vi "JKISM++ Post Message.vi"(8 "Error In (no error)":errorcluster, 9 "Dest Module":string="A", 10 "Arguments (\"\")":string, 11 "States":string="DoA") -> (0 "error IO":errorcluster)   [LabVIEW 2014, in "JKI-State-Machine-Plus.lvlib"]
uses:
  JKI-State-Machine-Plus.lvlib
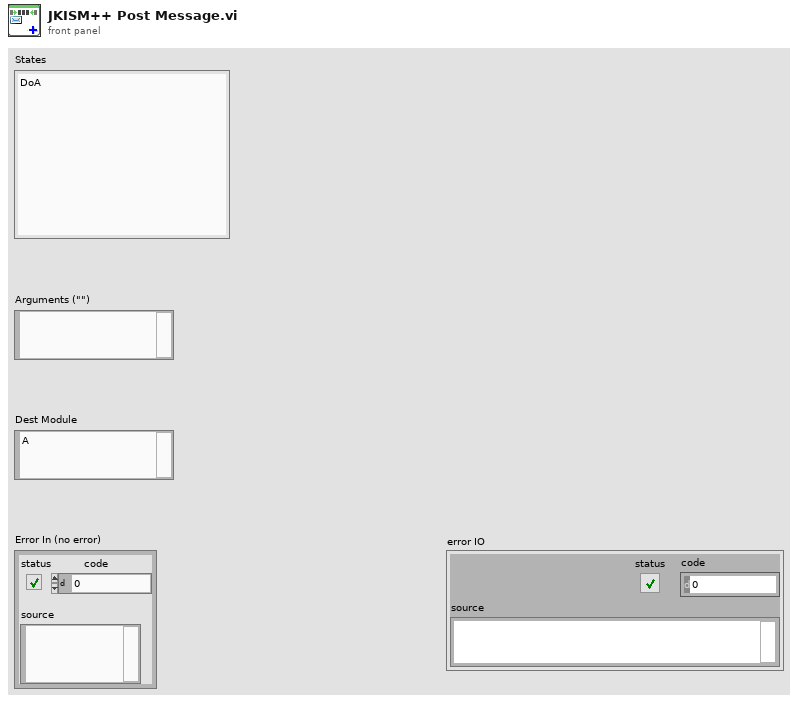
[diagram p1: front panel]
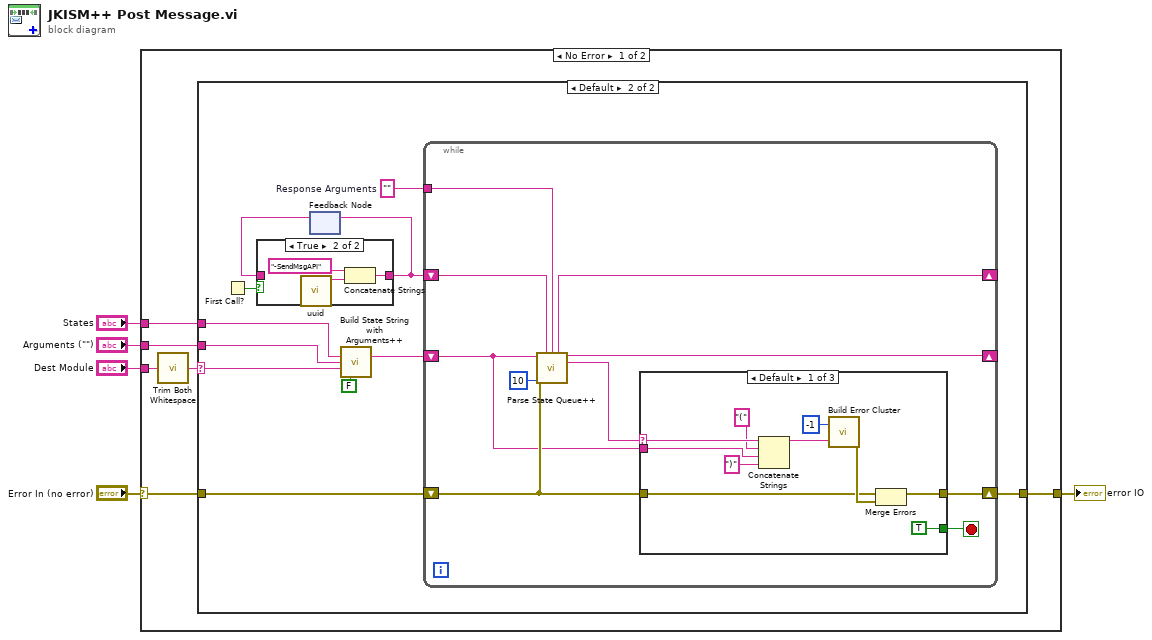
[diagram p0: block diagram]
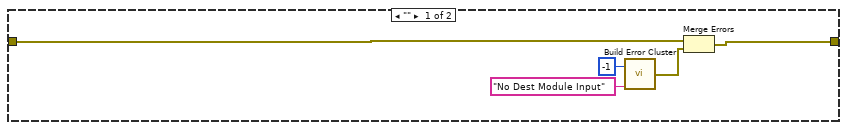
[diagram p2: hidden frame]
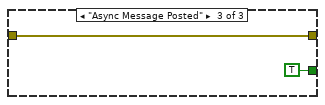
[diagram p5: hidden frame]
diagram:
  n1 = case shown="No Error" "Error In (no error)" {
    selector: "Error In (no error)" -> [w7 w55]
    tunnel: "States" -> [w11 _]
    tunnel: [w8 w55] -> w3
    tunnel: "Arguments (\"\")" -> [w10 _]
    tunnel: "Dest Module" -> [w9 _]
    frame No Error {
      n2 = call "Trim Both Whitespace.vi"("string"=w9) -> ("trimmed string"=w6:string)  [unwired: 1 in]
      n3 = case shown="Default" w6 {
        selector: w6 -> [_ w25]
        tunnel: w11 -> [_ w27]
        tunnel: w10 -> [_ w26]
        tunnel: [w15 w22] -> w8
        tunnel: w7 -> [w16 w21]
        frame "" {
          n4 = call "Build Error Cluster.vi"("String to Prepend to source (\"\")"="No Dest Module Input" ("String to Prepend to source (\"\")"), "code"=-1) -> ("error out"=w14:errorcluster)
          n5 = Merge Errors(w16, w14) -> (w15:errorcluster)
        }
        frame Default {
          w23 = ""  # Response Arguments
          n6 = First Call?() -> (First Call?: T/F=w19:bool)
          n7 = feedback #1() -> (w18:string)  [unwired: 1 in]
          n8 = case shown="True" w19 {
            tunnel: [w28 w29] -> w17
            tunnel: w18 -> [w28 _]
            frame False {
            }
            frame True {
              n9 = call "uuid.vi"() -> ("UUID"=w30:string)  [unwired: 11 in]
              n10 = Concatenate Strings("-SendMsgAPI" ("Name(\"\" to use uuid)"), w30) -> (w29:string)
            }
          }
          n11 = feedback-in #1(w17) -> ()
          n12 = call "Build State String with Arguments++.vi"("State"=w27, "Arguments (\"\")"=w26, "Dest Module (\"\")"=w25, "Sync-Call(@) T By Default/Async-Call(->) F"=FALSE) -> ("State with Arguments"=w20:string)  [unwired: 11 in]
          n13 = while {
            tunnel: w23 -> [w40]
            shift-right: [w38] -> w22
            shift-left: w21 -> [w37]
            shift-right: [w34] -> _
            shift-left: w20 -> [w35]
            shift-right: [w33] -> _
            shift-left: w17 -> [w36]
            stop <- w32 stop-if-true
            n14 = call "Parse State Queue++.vi"("State Queue"=w35, "Name(\"\" to use uuid)"=w36, "Response Arguments"=w40, "Error In (no error)"=w37, "Response Timeout(5000ms)"=10 ("Response Timeout(1000ms)")) -> ("Name Used"=w33:string, "Remaining States"=w34:string, "Current State"=w39:string)  [unwired: 5 in, 3 out]
            n15 = case shown="Default" w39 {
              selector: w39 -> [w50 _ _]
              tunnel: [w47 w52 w54] -> w38
              tunnel: w37 -> [w46 w52 w54]
              tunnel: w35 -> [w45 _ _]
              tunnel: [TRUE _ TRUE] -> w32
              frame Default {
                n16 = Concatenate Strings(w50, "(" ("string"), w45, ")" ("string")) -> (w49:string)
                n17 = call "Build Error Cluster.vi"("String to Prepend to source (\"\")"=w49, "code"=-1) -> ("error out"=w48:errorcluster)
                n18 = Merge Errors(w46, w48) -> (w47:errorcluster)
              }
              frame "Async Response" {
              }
              frame "Async Message Posted" {
              }
            }
          }
        }
      }
    }
    frame Error {
    }
  }
  "error IO" <- w3
